vi "GetRGBA.vi"(0 "ColorRGBA in":refnum<class "ColorRGBA.lvclass">, 11 "error in (no error)":errorcluster) -> (4 "ColorRGBA out":refnum<class "ColorRGBA.lvclass">, 6 "R":u8, 8 "G":u8, 10 "B":u8, 14 "A":u8, 15 "error out":errorcluster)   [LabVIEW 2021, in "Picture2D.lvlib" / "ColorRGBA.lvclass"]
uses:
  ColorRGBA.lvclass
  ColorRGBA.lvclass/ColorRGBA.ctl
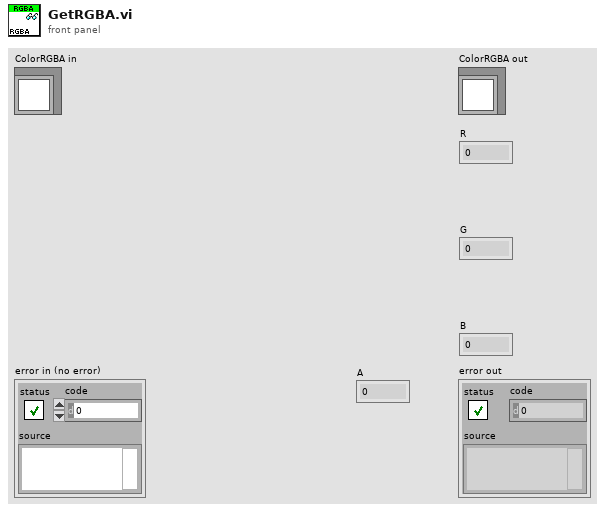
[diagram p1: front panel]
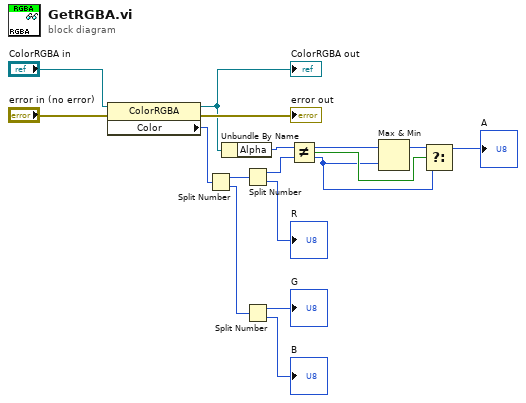
[diagram p0: block diagram]
diagram:
  n1 = property class="ColorRGBA"(reference="ColorRGBA in", error in="error in (no error)") -> (reference out=w6:refnum<class "ColorRGBA.lvclass">, error out=→"error out":errorcluster, "Color"=w14:u32)
  "ColorRGBA out" <- w6
  n2 = Split Number(x=w14) -> (hi(x)=w13:u16, lo(x)=w12:u16)
  n3 = Unbundle By Name(w6) -> ("Alpha"=w5:u8)
  n4 = Split Number(x=w13) -> (hi(x)=w1:u8, lo(x)=→"R":u8)
  n5 = Split Number(x=w12) -> (hi(x)=→"G":u8, lo(x)=→"B":u8)
  n6 = Not Equal?(x=w5, y=w1) -> (x != y?=w2:bool)
  n7 = Max & Min(x=w5, y=w1) -> (max(x,y)=w4:u8)  [unwired: 1 out]
  n8 = Select(t=w4, s=w2, f=w1) -> (s? t:f=→"A":u8)
